vi "Destroy.vi"(0 "reference in":refnum<class "BKP-911x Power Supply.lvclass">, 5 "error in (no error)":errorcluster) -> (14 "reference out":refnum<class "BKP-911x Power Supply.lvclass">, 19 "error out":errorcluster)   [LabVIEW 2018, in "BKP-911x Power Supply.lvclass"]
uses:
  BKP-911x Power Supply.lvclass
  <instrlib>/BK Precision 911X Series/BK Precision 911X Series.lvlib
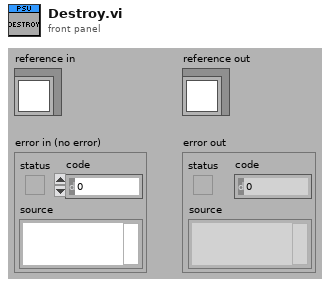
[diagram p1: front panel]
types:
  T1 = typedef "BKP-911x Power Supply.lvclass/ObjectAttributes.ctl" = cluster{"VISA resource name":refnum<visa-resource-name>, "Simulated?":bool, "Latest Values":dbl[], "Signal List":T2[], "Voltage Setpoint (V)":dbl, "Current Limit (A)":dbl, "Output Enabled?":bool}
  T2 = typedef "IO Signal List.ctl" = enum16{"Timestamp", "PSU_FB_U_VDC", "PSU_FB_I_AMP", "PSU_FB_W_WATT", "PSU_CMD_U_VDC", "PSU_CMD_I_AMP", "PSU_CMD_OUTPUT", "LCR_PRIMARY", "LCR_SECONDARY", "UV_R_Ohm", "UW_R_Ohm", "VW_R_Ohm", "UV_L_H", "UW_L_H", "VW_L_H", "U_U_VDC", "V_U_VDC", "W_U_VDC", "U_I_AMP", "V_I_AMP", "W_I_AMP", "PWM_CMD_DC_%", "PWM_CMD_VDC", "PWM_CMD_Hz", "PWM_FB_DC_%", "PWM_FB_VDC", "PWM_FB_Hz", "DO_RELAY_U_LCR_A", "DO_RELAY_V_LCR_A", "DO_RELAY_V_LCR_B", "DO_RELAY_W_LCR_B", "DIFF_UV_UW_L_H", "DIFF_UV_VW_L_H", "DIFF_UW_VW_L_H", "DIFF_UV_UW_R_Ohm", "DIFF_UV_VW_R_Ohm", "DIFF_UW_VW_R_Ohm", "DIFF_UV_U_VDC", "DIFF_UW_U_VDC", "DIFF_VW_U_VDC"}
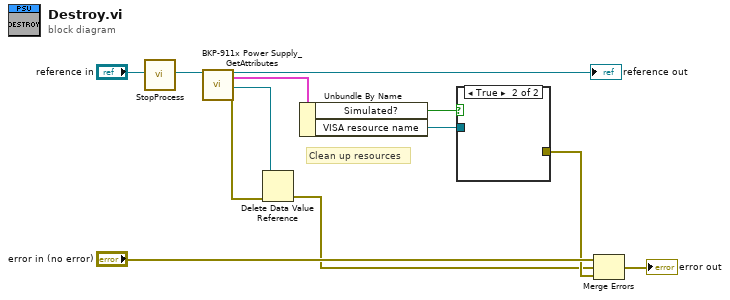
[diagram p0: block diagram]
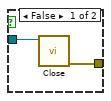
[diagram p2: hidden frame]
diagram:
  # "Clean up resources"
  n1 = call "StopProcess.vi"("reference in"="reference in") -> ("reference out"=w5:refnum<class "BKP-911x Power Supply.lvclass">)  [unwired: 17 in, 1 out]
  n2 = call "BKP-911x Power Supply_GetAttributes.vi"("reference in"=w5) -> ("reference out"=→"reference out":refnum<class "BKP-911x Power Supply.lvclass">, "Data"=w8:T1, "DataRef"=w9:refnum<data-value>, "error out"=w10:errorcluster)  [unwired: 15 in]
  n3 = Delete Data Value Reference(data value reference=w9, error in=w10) -> (error out=w2:errorcluster)  [unwired: 1 out]
  n4 = Unbundle By Name(w8) -> ("Simulated?"=w1:bool, "VISA resource name"=w3:refnum<visa-resource-name>)
  n5 = case shown="True" w1 {
    tunnel: [w14 _] -> w4
    tunnel: w3 -> [w13 _]
    frame False {
      n6 = call <instrlib>:"Close.vi"("VISA resource name"=w13) -> ("error out"=w14:errorcluster)  [unwired: 10 in]
    }
    frame True {
    }
  }
  n7 = Merge Errors("error in (no error)", w2, w4) -> (→"error out":errorcluster)
